vi "Request Address.vi"(0 "Destination Address":u8=255) -> (4 "Arb ID":u32 format="%.0x", 6 "Data":u8[](array[numeric]) format="%.0x")   [LabVIEW 2019, in "J1939 Utilities.lvlib"]
uses:
  J1939 Utilities.lvlib
  Request.vi
  Common Conversions.vi
  Convert J1939 ID to CAN Arb ID.vi
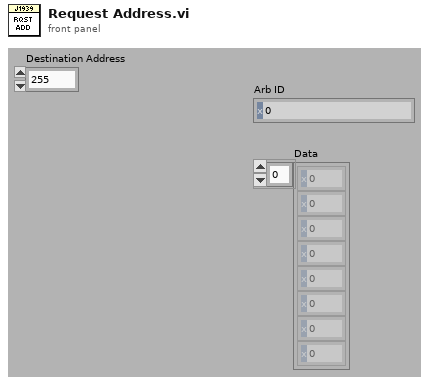
[diagram p1: front panel]
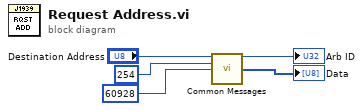
[diagram p0: block diagram]
diagram:
  n1 = call-poly "Common Messages.vi"("Destination Address"="Destination Address", "Source Address"=u8 254, "PGN"=u32 60928) -> ("Arb ID"=→"Arb ID":u32, "Data"=→"Data":u8[])  [unwired: 10 in, 1 out]
